vi "Delete Column.vi"(8 "error in":errorcluster, 9 "Column path":string, 10 "Table Path":string, 11 "LV-Data.PG":refnum<class "LV-Data.PGSQL.lvclass">) -> (0 "error out":errorcluster, 3 "LV-Data.PG out":refnum<class "LV-Data.PGSQL.lvclass">)   [LabVIEW 2016, in "LV-Data.PGSQL.lvclass"]
uses:
  LV-Data.PGSQL.lvclass
panel:
  out "Result":string[][](array[string])
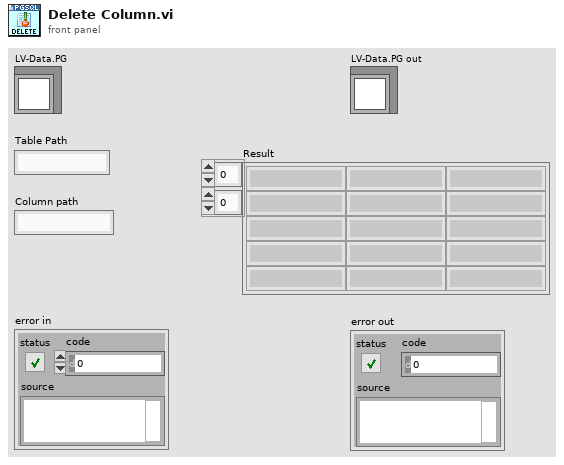
[diagram p1: front panel]
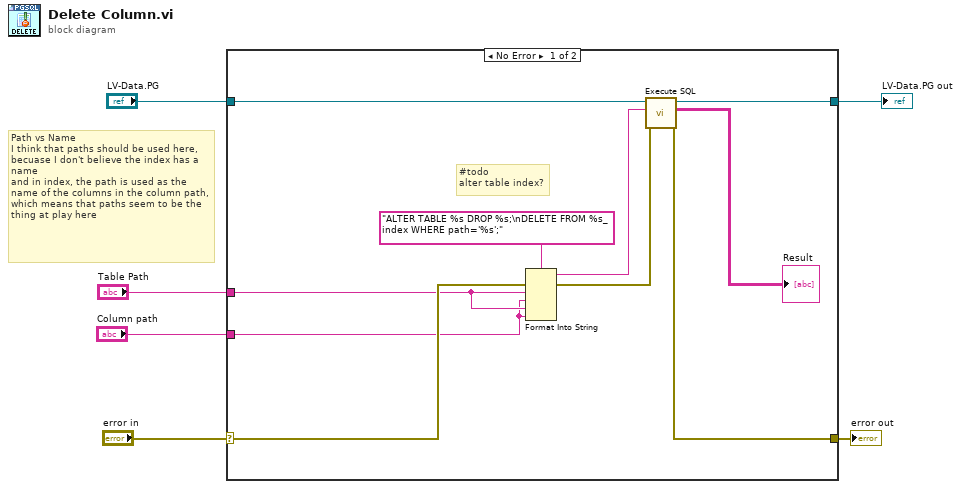
[diagram p0: block diagram]
diagram:
  # "Path vs Name\nI think that paths should be used here, becuase I don't believe the index has a name \nand in index, the path is used as the name of the columns in the column path, which means that paths seem to be the thing at play here"
  n1 = case shown="No Error" "error in" {
    selector: "error in" -> [w14 w18]
    tunnel: [w12 w18] -> w3
    tunnel: "Table Path" -> [w8 _]
    tunnel: "Column path" -> [w7 _]
    tunnel: "LV-Data.PG" -> [w11 w17]
    tunnel: [w10 w17] -> w1
    frame No Error {
      # "#todo\nalter table index?"
      n2 = Format Into String(format string="ALTER TABLE %s DROP %s;\nDELETE FROM %s_index WHERE path='%s';", error in=w14, w8, w7, w8, w7) -> (resulting string=w15:string, error out=w13:errorcluster)  [unwired: 1 in]
      n3 = call "Execute SQL.vi"("error in"=w13, "SQL"=w15, "LV-Data.PGSQL"=w11) -> ("error out"=w12:errorcluster, "Result"=→"Result":string[][], "LV-Data.PGSQL out"=w10:refnum<class "LV-Data.PGSQL.lvclass">)  [unwired: 6 in]
    }
    frame Error {
    }
  }
  "error out" <- w3
  "LV-Data.PG out" <- w1
